vi "Maxi Gauge-RW offset correction.vi"(0 "VISA-Ressource in":refnum<visa-resource-name>, 1 "Sensor 1 Set":i8(ring) items=["off", "on", "actual value"], 2 "Sensor 2 Set":i8(ring) items=["off", "on", "actual value"], 3 "Sensor 3 Set":i8(ring) items=["off", "on", "actual value"], 4 "Sensor 4 Set":i8(ring) items=["off", "on", "actual value"], 5 "Fehler (Eingang)":errorcluster, 6 "Node address":i8=-1 min=-1 max=31 step=1, 7 "Sensor 5 Set":i8(ring) items=["off", "on", "actual value"], 8 "W/R":bool, 9 "Sensor 6 Set":i8(ring) items=["off", "on", "actual value"]) -> (12 "Sensor 1 Get":i8(ring) items=["off", "on", "actual value"], 13 "Sensor 6 Get":i8(ring) items=["off", "on", "actual value"], 14 "VISA-Ressource out":refnum<visa-resource-name>, 15 "Sensor 2 Get":i8(ring) items=["off", "on", "actual value"], 16 "Sensor 3 Get":i8(ring) items=["off", "on", "actual value"], 17 "Sensor 4 Get":i8(ring) items=["off", "on", "actual value"], 18 "Sensor 5 Get":i8(ring) items=["off", "on", "actual value"], 19 "Fehler (Ausgang)":errorcluster)   [LabVIEW 2012, in "Maxi Gauge.lvlib"]
uses:
  Maxi Gauge.lvlib
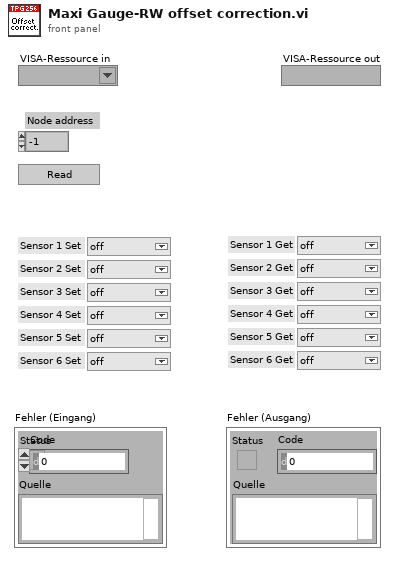
[diagram p1: front panel]
types:
  T1 = cluster{"[0]":i8, "[1]":i8, "[2]":i8, "[3]":i8, "[4]":i8, "[5]":i8}
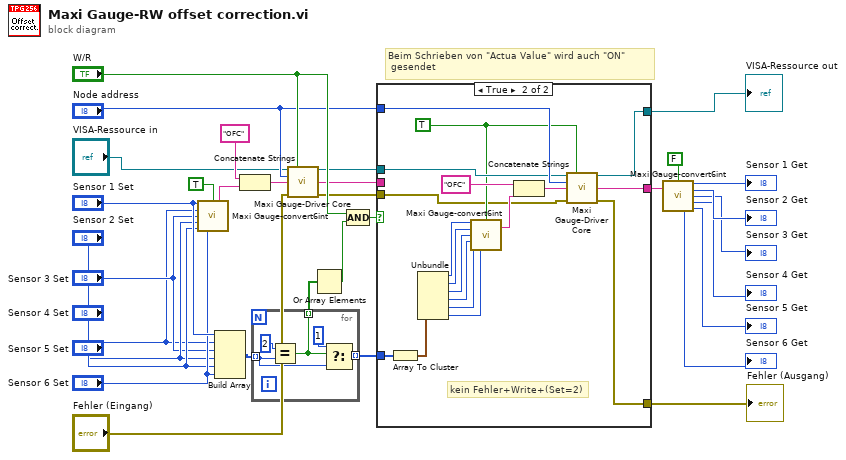
[diagram p0: block diagram]
diagram:
  # "Beim Schrieben von \"Actua Value\" wird auch \"ON\"\n gesendet"
  n1 = call "Maxi Gauge-convert6int.vi"("Integer1 in"="Sensor 1 Set", "W/R [W: Int in; Str out ]"=TRUE, "Integer2 in"="Sensor 2 Set", "Integer3 in"="Sensor 3 Set", "Integer4 in"="Sensor 4 Set", "Integer5 in"="Sensor 5 Set", "Integer6 in"="Sensor 6 Set") -> ("String out"=w16:string)  [unwired: 2 in, 6 out]
  n2 = Build Array("Sensor 1 Set", "Sensor 2 Set", "Sensor 3 Set", "Sensor 4 Set", "Sensor 5 Set", "Sensor 6 Set") -> (w12:i8[])
  n3 = Concatenate Strings("OFC", w16) -> (w6:string)
  n4 = for {
    tunnel: w12 -> [w36] mode=indexing
    tunnel: [w34] -> w11 mode=indexing
    tunnel: [w33] -> w8 mode=indexing
    n5 = Equal?(x=i8 2, y=w36) -> (x = y?=w34:bool)
    n6 = Select(t=i8 1, s=w34, f=w36) -> (s? t:f=w33:i8)
  }
  n7 = call "Maxi Gauge-Driver Core.vi"("VISA-Ressource in"="VISA-Ressource in", "Write/Read"="W/R", "Node address"="Node address", "Command"=w6, "Fehler (Eingang)"="Fehler (Eingang)") -> ("VISA-Ressource out"=w3:refnum<visa-resource-name>, "String Out"=w14:string, "Fehler (Ausgang)"=w7:errorcluster)  [unwired: 8 in]
  n8 = Or Array Elements(Boolean array=w11) -> (logical OR=w10:bool)
  n9 = Compound Arithmetic op=AND("W/R", w10) -> (w13:bool)
  n10 = case shown="True" w13 {
    tunnel: w14 -> [w40 _]
    tunnel: [w40 w47] -> w9
    tunnel: w8 -> [_ w58]
    tunnel: "Node address" -> [_ w48]
    tunnel: [w39 w46] -> w5
    tunnel: w7 -> [w39 w41]
    tunnel: w3 -> [w38 w44]
    tunnel: [w38 w43] -> w2
    frame False {
    }
    frame True {
      w42 = TRUE ("W/R [W: Int in; Str out ]")
      # "kein Fehler+Write+(Set=2)"
      n11 = Array To Cluster(array=w58) -> (cluster=w57:T1)
      n12 = Unbundle(w57) -> ("[0]"=w54:i8, "[1]"=w53:i8, "[2]"=w52:i8, "[3]"=w51:i8, "[4]"=w50:i8, "[5]"=w49:i8)
      n13 = call "Maxi Gauge-convert6int.vi"("Integer1 in"=w54, "W/R [W: Int in; Str out ]"=w42, "Integer2 in"=w53, "Integer3 in"=w52, "Integer4 in"=w51, "Integer5 in"=w50, "Integer6 in"=w49) -> ("String out"=w55:string)  [unwired: 2 in, 6 out]
      n14 = Concatenate Strings("OFC", w55) -> (w45:string)
      n15 = call "Maxi Gauge-Driver Core.vi"("VISA-Ressource in"=w44, "Write/Read"=w42, "Node address"=w48, "Command"=w45, "Fehler (Eingang)"=w41) -> ("VISA-Ressource out"=w43:refnum<visa-resource-name>, "String Out"=w47:string, "Fehler (Ausgang)"=w46:errorcluster)  [unwired: 8 in]
    }
  }
  "Fehler (Ausgang)" <- w5
  "VISA-Ressource out" <- w2
  n16 = call "Maxi Gauge-convert6int.vi"("String in"=w9, "W/R [W: Int in; Str out ]"=FALSE) -> ("Integer1 out"=→"Sensor 1 Get":u8, "Integer2 out"=→"Sensor 2 Get":u8, "Integer3 out"=→"Sensor 3 Get":u8, "Integer4 out"=→"Sensor 4 Get":u8, "Integer6 out"=→"Sensor 6 Get":u8, "Integer5 out"=→"Sensor 5 Get":u8)  [unwired: 7 in, 1 out]
